vi "窗口弹出对话框(子VI).vi"(11 "消息":string) -> (3 "true":bool)   [LabVIEW 2016, in "斯坦道CODMn.lvlib"]
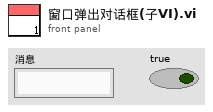
[diagram p1: front panel]
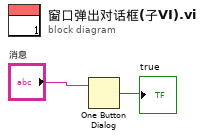
[diagram p0: block diagram]
diagram:
  n1 = One Button Dialog(message="消息") -> (true=→"true":bool)  [unwired: 1 in]
